vi "Create_Error_log_folders.vi"(3 "Per Day Log File?":bool, 4 "Log Folder":string, 5 "Log Filename":string) -> (0 "exists?":bool, 1 "Server copy Location":path, 2 "Local Log File":path)   [LabVIEW 2014]
uses:
  Globals/Constants_global.vi
  Globals/Preference_global.vi
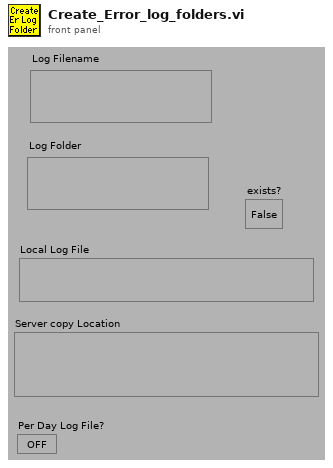
[diagram p1: front panel]
types:
  T1 = cluster{"second":i32, "minute":i32, "hour":i32, "day of month":i32, "month":i32, "year":i32, "day of week":i32, "day of year":i32, "is DST":i32}
  T2 = typedef "EnFlo_Data_Folder_Setup.ctl" = string
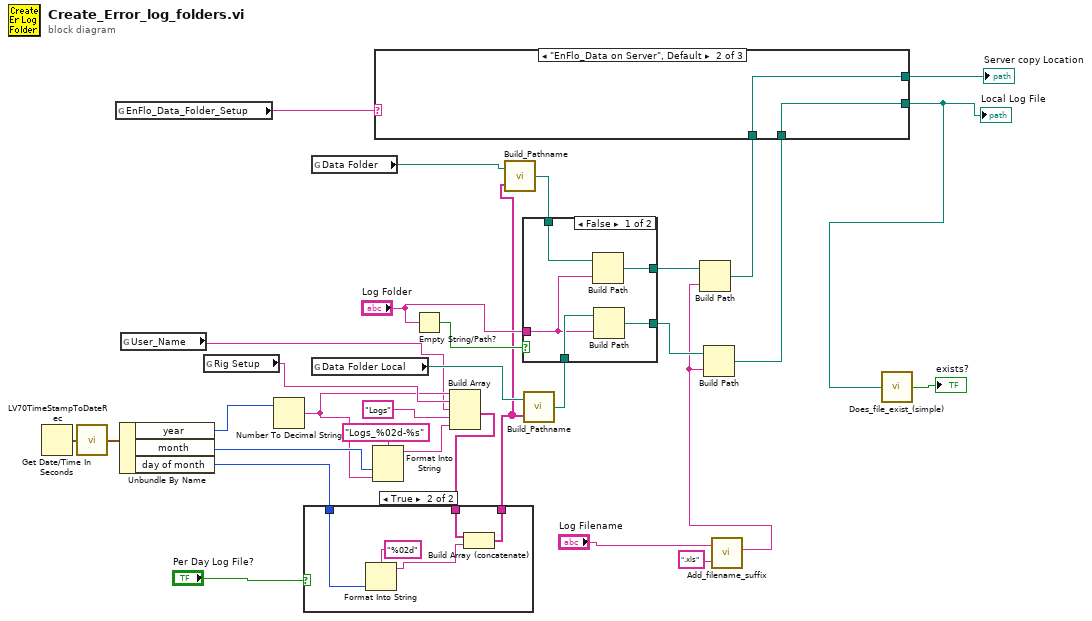
[diagram p0: block diagram]
diagram:
  n1 = Get Date/Time In Seconds() -> (seconds since 1Jan1904=w7:timestamp)
  n2 = call <vilib>:"LV70TimeStampToDateRec.vi"("time stamp"=w7) -> ("date time rec"=w30:T1)
  n3 = global read "Preference_global.vi" "EnFlo_Data_Folder_Setup"() -> (w5:T2)
  n4 = Unbundle By Name(w30) -> ("year"=w29:i32, "month"=w21:i32, "day of month"=w10:i32)
  n5 = global read "Preference_global.vi" "User_Name"() -> (w6:string)
  n6 = global read "Preference_global.vi" "Rig Setup"() -> (w23:string)
  n7 = Number To Decimal String(number=w29) -> (decimal integer string=w20:string)  [unwired: 1 out]
  n8 = global read "Constants_global.vi" "Data Folder"() -> (w15:path)
  n9 = global read "Constants_global.vi" "Data Folder Local"() -> (w28:path)
  n10 = Format Into String(format string="Logs_%02d-%s", w21, w20) -> (resulting string=w18:string)  [unwired: 2 in, 1 out]
  n11 = Empty String/Path?(string/path="Log Folder") -> (empty?=w24:bool)
  n12 = Build Array(w20, w23, w6, "Logs", w18) -> (w9:string[])
  n13 = case shown="True" "Per Day Log File?" {
    tunnel: w10 -> [_ w36]
    tunnel: w9 -> [w32 w34]
    tunnel: [w32 w33] -> w8
    frame False {
    }
    frame True {
      n14 = Format Into String(format string="%02d", w36) -> (resulting string=w35:string)  [unwired: 2 in, 1 out]
      n15 = Build Array (concatenate)(w34, w35) -> (w33:string[])
    }
  }
  n16 = call "Build_Pathname.vi"("PathElements"=w8, "PathnameIn"=w15) -> ("AppendedPath"=w14:path)
  n17 = call "Build_Pathname.vi"("PathElements"=w8, "PathnameIn"=w28) -> ("AppendedPath"=w26:path)
  n18 = case shown="False" w24 {
    tunnel: w26 -> [w42 w44]
    tunnel: [w41 w44] -> w31
    tunnel: "Log Folder" -> [w39 _]
    tunnel: w14 -> [w40 w43]
    tunnel: [w38 w43] -> w13
    frame False {
      n19 = Build Path(base path=w40, name or relative path=w39) -> (appended path=w38:path)
      n20 = Build Path(base path=w42, name or relative path=w39) -> (appended path=w41:path)
    }
    frame True {
    }
  }
  n21 = call "Add_filename_suffix.vi"("Filename"="Log Filename", "Suffix to add"=".xls") -> ("Filename out"=w12:string)  [unwired: 3 out]
  n22 = Build Path(base path=w13, name or relative path=w12) -> (appended path=w3:path)
  n23 = Build Path(base path=w31, name or relative path=w12) -> (appended path=w2:path)
  n24 = case shown="\"EnFlo_Data on Server\", Default" w5 {
    tunnel: [w45 w47 w48] -> w4
    tunnel: w3 -> [w45 w47 w48]
    tunnel: [w45 w46 w48] -> w1
    tunnel: w2 -> [_ w46 _]
    frame "EnFlo_Data on C drive - do not backup" {
    }
    frame "EnFlo_Data on Server", Default {
    }
    frame "EnFlo_Data on C drive - backup to server" {
    }
  }
  "Local Log File" <- w1
  "Server copy Location" <- w4
  n25 = call "Does_file_exist_(simple).vi"("Pathname"=w1) -> ("exists?"=→"exists?":bool)
